vi "Video snapshot.vi"(1 "Image name":string="test", 2 "Image directory path":path=path "C:/test", 3 "VideoMode":u32, 4 "Interface name":T1="cam0") -> (0 "Error Out":errorcluster)   [LabVIEW 2014]
uses:
  <vilib>/userdefined/High Color/IMAQdx.ctl
  <vilib>/vision/driver/IMAQdx.llb/IMAQdx Camera Control Mode.ctl
  <vilib>/vision/driver/NI_Vision_Acquisition_Software.lvlib
  <resource>/objmgr/imaqdx.rc
panel:
  out "Image":T2(plugin-control)
  # "PN 27/11/2014"
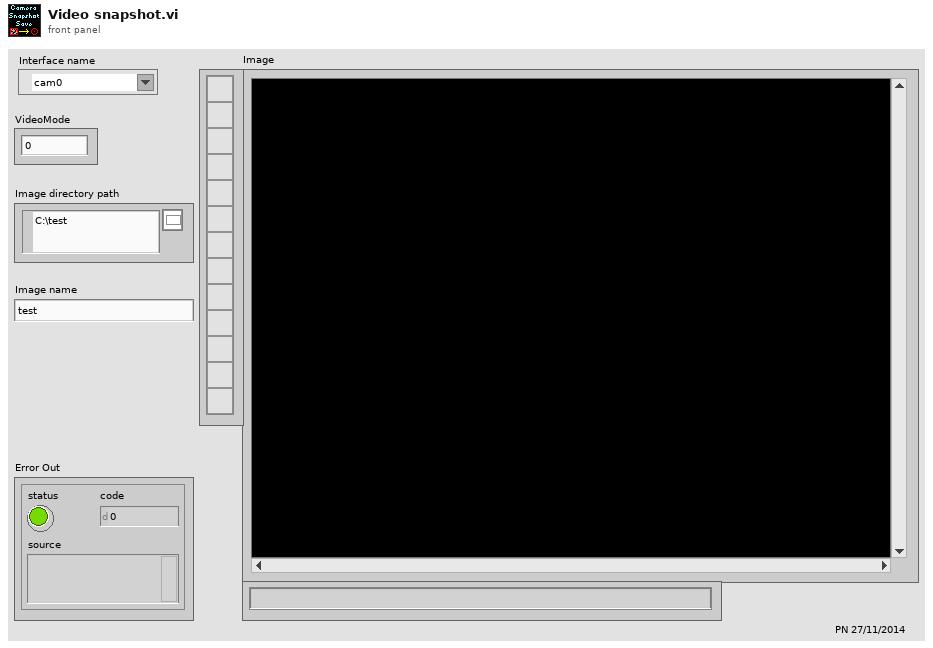
[diagram p1: front panel]
types:
  T1 = typedef "IMAQdx.ctl" = refnum<k21>
  T2 = typedef "IMAQ Image.ctl" = refnum<image>
  T3 = typedef "Image Type" = u32
  T4 = typedef "NI_Vision_Acquisition_Software.lvlib/IMAQdx Camera Control Mode.ctl" = enum32{"Controller", "Listener"}
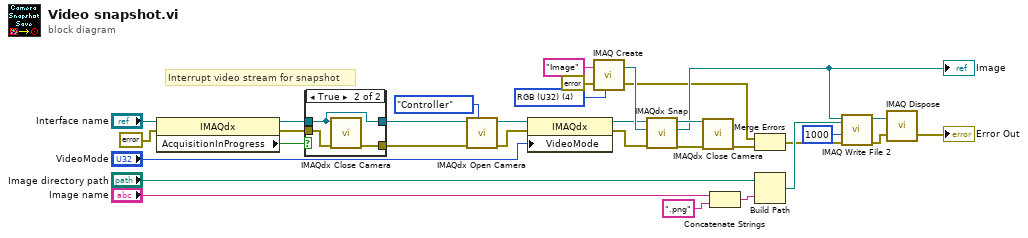
[diagram p0: block diagram]
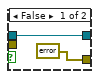
[diagram p2: hidden frame]
diagram:
  w18 = T3 4 items=["Grayscale (U8)", "Grayscale (I16)", "Grayscale (SGL)", "Complex (CSG)", "RGB (U32)", "HSL (U32)", "RGB (U64)", "Grayscale (U16)"] ("Image Type")
  # "Interrupt video stream for snapshot"
  n1 = property class="IMAQdx"(reference="Interface name", error in=errorcluster {"status"=FALSE, "code"=0, "source"=""}) -> (reference out=w6:T1, error out=w5:errorcluster, "AcquisitionInProgress"=w7:bool)
  n2 = case shown="True" w7 {
    tunnel: w6 -> [w34 w35]
    tunnel: w5 -> [_ w37]
    tunnel: [errorcluster {"status"=FALSE, "code"=0, "source"=""} ("error in") w36] -> w4
    tunnel: [w34 w35] -> w3
    frame False {
    }
    frame True {
      n3 = call <vilib>:"IMAQdx Close Camera.vi"("error in"=w37, "Session In"=w35) -> ("error out"=w36:errorcluster)  [unwired: 9 in]
    }
  }
  n4 = call <vilib>:"IMAQdx Open Camera.vi"("Camera Control Mode"=IMAQdx_Camera_Control_Mode."Controller", "error in"=w4, "Session In"=w3) -> ("error out"=w11:errorcluster, "Session Out"=w13:T1)  [unwired: 7 in]
  n5 = property class="IMAQdx"(reference=w13, error in=w11, "VideoMode"="VideoMode") -> (reference out=w12:T1, error out=w10:errorcluster)
  n6 = call "IMAQ Create"("Image Name"="Image", "Image Type"=w18, "error in (no error)"=errorcluster {"status"=FALSE, "code"=0, "source"=""} ("error in")) -> ("New Image"=w29:T2, "error out"=w16:errorcluster)  [unwired: 2 in]
  n7 = call <vilib>:"IMAQdx Snap.vi"("error in"=w10, "Image In"=w29, "Session In"=w12) -> ("error out"=w31:errorcluster, "Image Out"=w27:T2, "Session Out"=w32:T1)  [unwired: 6 in]
  "Image" <- w27
  n8 = call <vilib>:"IMAQdx Close Camera.vi"("error in"=w31, "Session In"=w32) -> ("error out"=w15:errorcluster)  [unwired: 9 in]
  n9 = Concatenate Strings("Image name", ".png" ("name or relative path")) -> (w21:string)
  n10 = Merge Errors(w16, w15) -> (w17:errorcluster)
  n11 = Build Path(base path="Image directory path", name or relative path=w21) -> (appended path=w20:path)
  n12 = call-poly "IMAQ Write File 2"("error in (no error)"=w17, "Image Quality"=u32 1000, "File Path"=w20, "Image"=w27) -> ("error out"=w25:errorcluster, "Image Out (duplicate)"=w26:T2)  [unwired: 6 in]
  n13 = call "IMAQ Dispose"("Image"=w26, "error in (no error)"=w25) -> ("error out"=→"Error Out":errorcluster)  [unwired: 4 in]
